vi "resetboard.vi"(8 "error in (no error)":errorcluster, 10 "address":string, 11 "remote port or service name":u16=9764) -> (0 "error out":errorcluster, 3 "Data out":string)   [LabVIEW 2009]
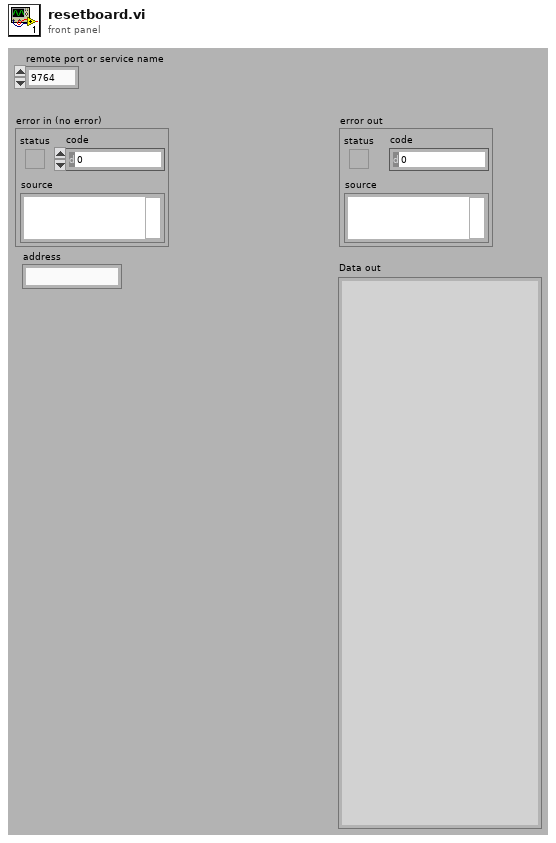
[diagram p1: front panel]
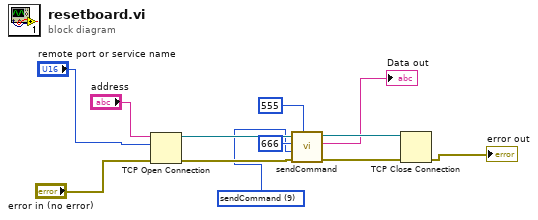
[diagram p0: block diagram]
diagram:
  w5 = u16 9 items=["sendCommand"=9, "FPGA_writeRegister"=3, "FPGA_readRegister"=2, "uC_writeRegister"=1, "uC_readRegister"=0] ("Action")
  n1 = TCP Open Connection(address="address", remote port or service name="remote port or service name", error in (no error)="error in (no error)") -> (connection ID=w9:refnum<k5>, error out=w12:errorcluster)  [unwired: 2 in]
  n2 = call "sendCommand.vi"("Data"=555, "error in"=w12, "Action"=w5, "id_in"=666, "connection ID"=w9) -> ("error out"=w11:errorcluster, "Data out"=→"Data out":string, "connection ID out"=w8:refnum<k5>)  [unwired: 2 in, 2 out]
  n3 = TCP Close Connection(connection ID=w8, error in (no error)=w11) -> (error out=→"error out":errorcluster)  [unwired: 1 in, 1 out]
